vi "MoveAbsSingleAxis.vi"(6 "Wait":bool=TRUE, 8 "error in (no error)":errorcluster, 9 "Value":dbl format="%.2f", 10 "Axis":i32=1, 11 "DelayLineSimulation in":refnum<class "DelayLineEmulate.lvclass">) -> (0 "error out":errorcluster, 3 "DelayLineSimulation out":refnum<class "DelayLineEmulate.lvclass">)   [LabVIEW 2015, in "DelayLineEmulate.lvclass"]
uses:
  DelayLineEmulate.lvclass
  DelayLine.lvclass/DelayLine.ctl
  DelayLine.lvclass
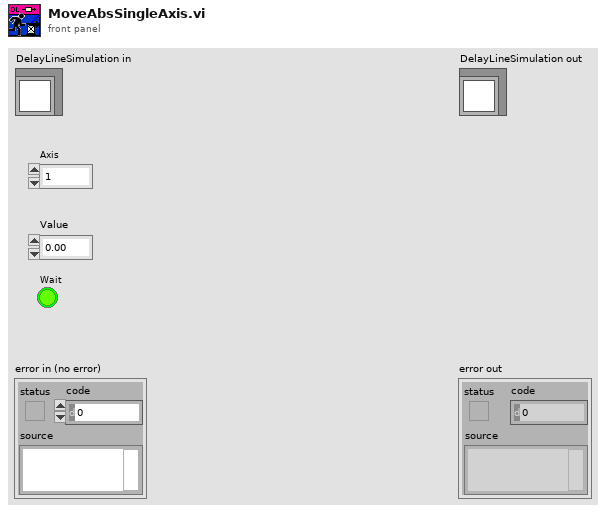
[diagram p1: front panel]
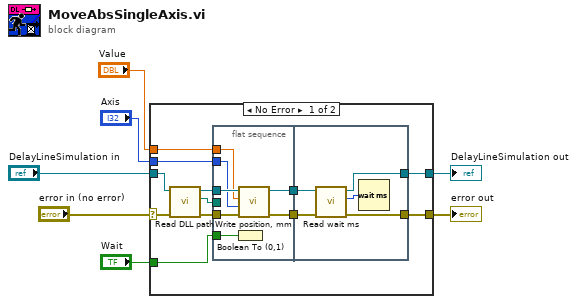
[diagram p0: block diagram]
diagram:
  n1 = case shown="No Error" "error in (no error)" {
    selector: "error in (no error)" -> [w19 w33]
    tunnel: [w10 w33] -> w3
    tunnel: "Value" -> [w14 _]
    tunnel: "Axis" -> [w13 _]
    tunnel: "Wait" -> [w12 _]
    tunnel: "DelayLineSimulation in" -> [w11 w32]
    tunnel: [w9 w32] -> w1
    frame No Error {
      n2 = call "Read DLL path.vi"("error in (no error)"=w19, "DelayLine in"=w11) -> ("error out"=w18:errorcluster, "DLL path"=w17:path, "DelayLine out"=w16:refnum<class "DelayLineEmulate.lvclass">)  [unwired: 7 in]
      n3 = flat-sequence {
        tunnel: w18 -> [w24]
        tunnel: w17 -> [_]
        tunnel: w16 -> [w25]
        tunnel: [w22] -> w15
        tunnel: w14 -> [w21]
        tunnel: w13 -> [w20]
        tunnel: w12 -> [w26]
        tunnel: [w23] -> w8
        tunnel: w15 -> [w31]
        tunnel: [w29] -> w10
        tunnel: [w28] -> w9
        tunnel: w8 -> [w27]
        frame #0 {
          n4 = Boolean To (0,1)(Boolean=w26) -> ()  [unwired: 1 out]
          n5 = call "Write position, mm.vi"("error in (no error)"=w24, "axis"=w20, "position, mm"=w21, "DelayLineSimulation in"=w25) -> ("error out"=w23:errorcluster, "DelayLineSimulation out"=w22:refnum<class "DelayLineEmulate.lvclass">)  [unwired: 6 in]
        }
        frame #1 {
          n6 = call "Read wait ms.vi"("error in (no error)"=w27, "DelayLine in"=w31) -> ("error out"=w29:errorcluster, "wait ms"=w30:i32, "DelayLine out"=w28:refnum<class "DelayLineEmulate.lvclass">)  [unwired: 7 in]
          n7 = Wait (ms)(milliseconds to wait=w30) -> ()  [unwired: 1 out]
        }
      }
    }
    frame Error {
    }
  }
  "error out" <- w3
  "DelayLineSimulation out" <- w1
